vi "BuildTileCodes.vi"(9 "CameraPos":T1, 10 "Position":T1, 11 "TileCodes":u32[][](array[numeric])) -> (3 "Array":u64[](array[numeric]))   [LabVIEW 2019, in "RT_Game.lvlib" / "Engine.lvclass"]
uses:
  Engine.lvclass
  Game/Coordinate.ctl
  Game/Game.lvclass
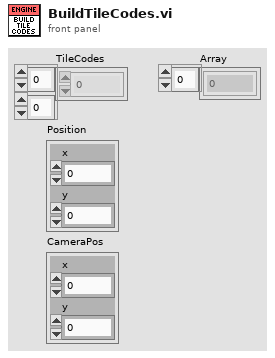
[diagram p1: front panel]
types:
  T1 = typedef "RT_Game.lvlib/Game.lvclass/Coordinate.ctl" = cluster{"x":dbl, "y":dbl}
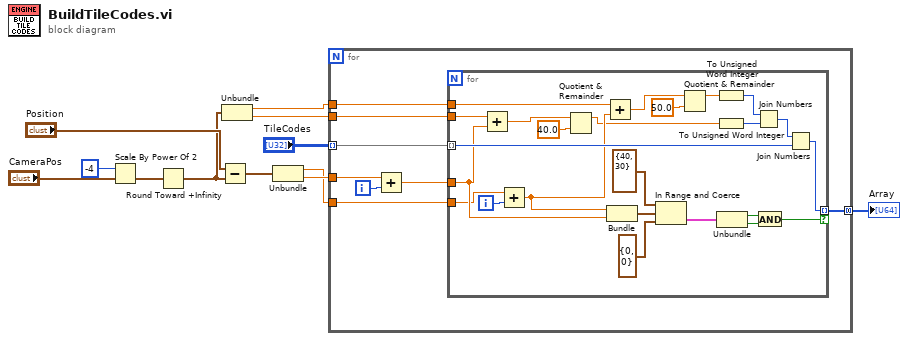
[diagram p0: block diagram]
diagram:
  n1 = Scale By Power Of 2(n=i16 -4, x="CameraPos") -> (x*2^n=w3:T1)
  n2 = Round Toward +Infinity(x=w3) -> (ceil(x): smallest int >= x=w1:T1)
  n3 = Subtract(x="Position", y=w1) -> (x-y=w9:T1)
  n4 = Unbundle(w1) -> ("x"=w5:dbl, "y"=w4:dbl)
  n5 = Unbundle(w9) -> ("x"=w7:dbl, "y"=w8:dbl)
  n6 = for {
    tunnel: [w19] -> w12 mode=concatenating
    tunnel: "TileCodes" -> [w18] mode=indexing
    tunnel: w8 -> [w17]
    tunnel: w7 -> [w16]
    tunnel: w5 -> [w15]
    tunnel: w4 -> [w14]
    i -> [w20]
    n7 = Add(x=w17, y=w20) -> (x+y=w13:dbl)
    n8 = for {
      tunnel: w13 -> [w40]
      tunnel: [w43] -> w19 mode=indexing if=w35
      tunnel: w18 -> [w41] mode=indexing
      tunnel: w16 -> [w31]
      tunnel: w15 -> [w28]
      tunnel: w14 -> [w27]
      i -> [w44]
      n9 = Add(x=w27, y=w40) -> (x+y=w29:dbl)
      n10 = Add(x=w31, y=w44) -> (x+y=w32:dbl)
      n11 = Quotient & Remainder(x=w29, y=40.0 ("x")) -> (x-y*floor(x/y)=w24:dbl)  [unwired: 1 out]
      n12 = Add(x=w28, y=w32) -> (x+y=w30:dbl)
      n13 = Bundle(w32, w40) -> (w39:cluster{dbl, dbl})  [unwired: 1 in]
      n14 = In Range and Coerce(upper limit=cluster{u16, u16} {40, 30}, x=w39, lower limit=cluster{u16, u16} {0, 0}) -> (In Range?=w36:cluster{bool, bool})  [unwired: 1 out]
      n15 = Quotient & Remainder(x=w30, y=50.0 ("x")) -> (x-y*floor(x/y)=w23:dbl)  [unwired: 1 out]
      n16 = To Unsigned Word Integer(number=w23) -> (unsigned 16bit integer=w22:u16)
      n17 = To Unsigned Word Integer(number=w24) -> (unsigned 16bit integer=w21:u16)
      n18 = Unbundle(w36) -> (w37:bool, w38:bool)
      n19 = Join Numbers(hi=w22, lo=w21) -> ((hi.lo)=w42:u32)
      n20 = And(x=w37, y=w38) -> (x .and. y?=w35:bool)
      n21 = Join Numbers(hi=w42, lo=w41) -> ((hi.lo)=w43:u64)
    }
  }
  "Array" <- w12
